vi "Update Robot Pose.vi"(10 "x_k|k":T2, 11 "Detection Robot in":T1 {"height" format="%+4.3f"; "pixel_y" format="%+4.3f"; "pixel_x" format="%+4.3f"; "orientation" format="%+4.3f"; "y" format="%+4.3f"; "confidence" format="%4.3f"; "x" format="%+4.3f"}) -> (3 "Detection Robot out":T1 {"height" format="%+4.3f"; "pixel_y" format="%+4.3f"; "pixel_x" format="%+4.3f"; "orientation" format="%+4.3f"; "y" format="%+4.3f"; "confidence" format="%4.3f"; "x" format="%+4.3f"})   [LabVIEW 2018]
uses:
  <vilib>/Analysis/Matrix/Datatypes/RealMatrix.ctl
  git/SSLView/SSL Detection Robot.ctl
  <vilib>/Analysis/Matrix/NI_Matrix.lvlib
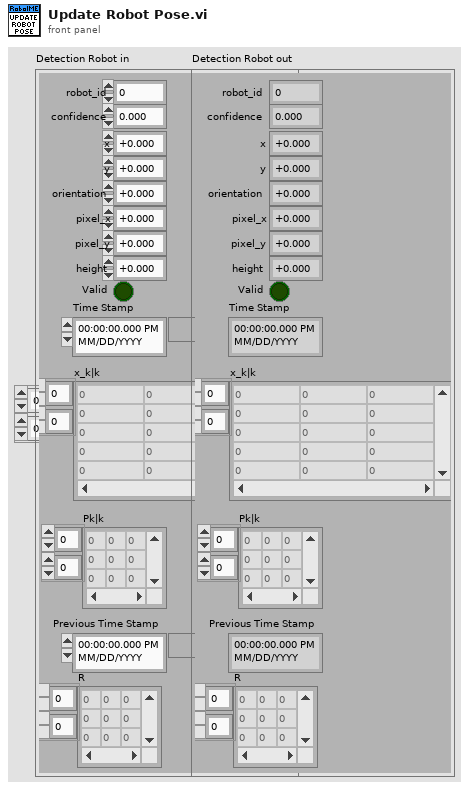
[diagram p1: front panel]
types:
  T1 = typedef "SSL Detection Robot.ctl" = cluster{"x":sgl, "robot_id":u32, "confidence":sgl, "y":sgl, "orientation":sgl, "pixel_x":sgl, "pixel_y":sgl, "height":sgl, "Valid":bool, "Time Stamp":timestamp, "x_k|k":T2, "Pk|k":T2, "Previous Time Stamp":timestamp, "R":T2}
  T2 = typedef "NI_Matrix.lvlib/RealMatrix.ctl" = dbl[][]
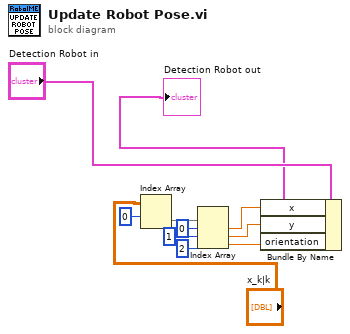
[diagram p0: block diagram]
diagram:
  n1 = Index Array(array="x_k|k", index (row)=0) -> (element=w4:dbl[])  [unwired: 1 in]
  n2 = Index Array(array=w4, index #1=0 ("index"), index #2=1 ("index"), index #3=2 ("index")) -> (element #1=w5:dbl, element #2=w6:dbl, element #3=w7:dbl)
  n3 = Bundle By Name(cluster="Detection Robot in", "x"=w5, "y"=w6, "orientation"=w7) -> (→"Detection Robot out":T1)
